vi "init.vi"(8 "error in (no error)":errorcluster, 11 "Input":string="34,45,89") -> (0 "error out":errorcluster, 3 "Output":string)   [LabVIEW 2019]
panel:
  # "."
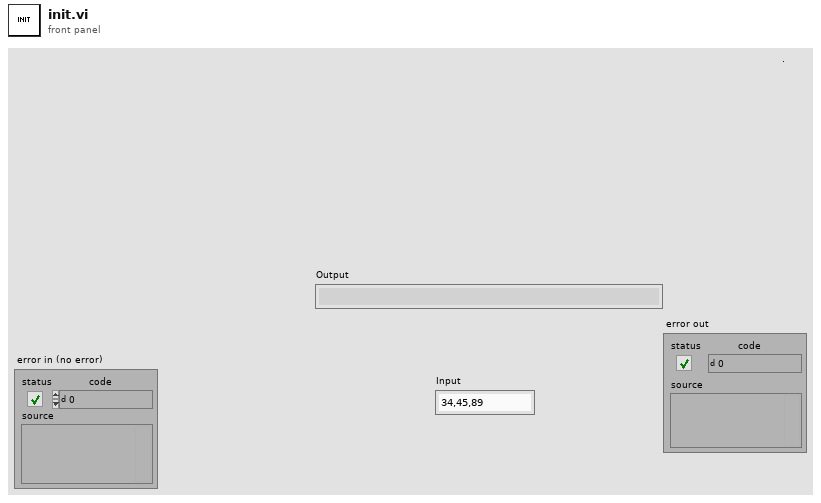
[diagram p1: front panel]
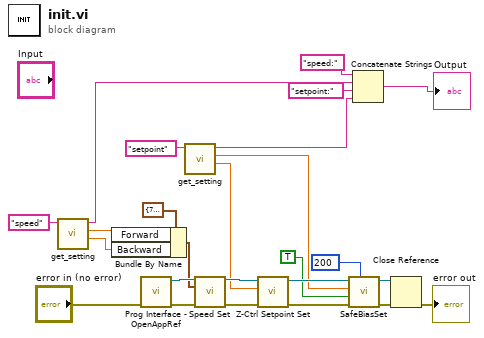
[diagram p0: block diagram]
diagram:
  n1 = call "get_setting.vi"("key"="speed") -> ("output 2"=w1:dbl, "output 1"=w2:dbl, "value"=w5:string)  [unwired: 6 in, 2 out]
  n2 = Bundle By Name(cluster=cluster{"Forward":sgl, "Backward":sgl} {"Forward"=8e-08, "Backward"=1.6e-07} ("Speed (m/s)"), "Forward"=w2, "Backward"=w1) -> (w12:cluster{"Forward":sgl, "Backward":sgl})
  n3 = call <userlib>:"Prog Interface - OpenAppRef.vi"("Error in (no error)"="error in (no error)") -> ("Error out"=w22:errorcluster, "Application reference"=w23:refnum<vi>)  [unwired: 5 in]
  n4 = call "get_setting.vi"("key"="setpoint") -> ("output 2"=w3:dbl, "output 1"=w4:dbl, "value"=w6:string)  [unwired: 6 in, 2 out]
  n5 = call <userlib>:"Speed Set.vi"("Application ref in"=w23, "Speed (m/s)"=w12, "error in (no error)"=w22) -> ("Application ref out"=w17:refnum<vi>, "error out"=w21:errorcluster)  [unwired: 11 in]
  n6 = call <userlib>:"Z-Ctrl Setpoint Set.vi"("error in (no error)"=w21, "Z Controller setpoint"=w3, "Application ref in"=w17) -> ("error out"=w20:errorcluster, "Application ref out"=w16:refnum<vi>)  [unwired: 7 in]
  n7 = call "SafeBiasSet.vi"("Application ref in"=w16, "Bias (V)"=w4, "Ramp"=TRUE, "error in (no error)"=w20, "milliseconds to wait"=u32 200) -> ("Application ref out"=w19:refnum<vi>, "Error out"=w18:errorcluster)  [unwired: 4 in]
  n8 = Concatenate Strings("speed:" ("string"), w5, "setpoint:" ("string"), w6) -> (→"Output":string)
  n9 = Close Reference(reference=w19, error in (no error)=w18) -> (error out=→"error out":errorcluster)
